vi "Write cmd queue ref.vi"(8 "error in (no error)":errorcluster, 10 "cmd queue":refnum<queue>, 11 "Plots in":refnum<class "Plots.lvclass">) -> (0 "error out":errorcluster, 3 "Plots out":refnum<class "Plots.lvclass">)   [LabVIEW 2017, in "Plots.lvclass"]
doc: "writes the reference of the commands queue to the private property. the queue is used to share data between scripts and plots."
uses:
  Plots.lvclass
  Plots.lvclass/Plots.ctl
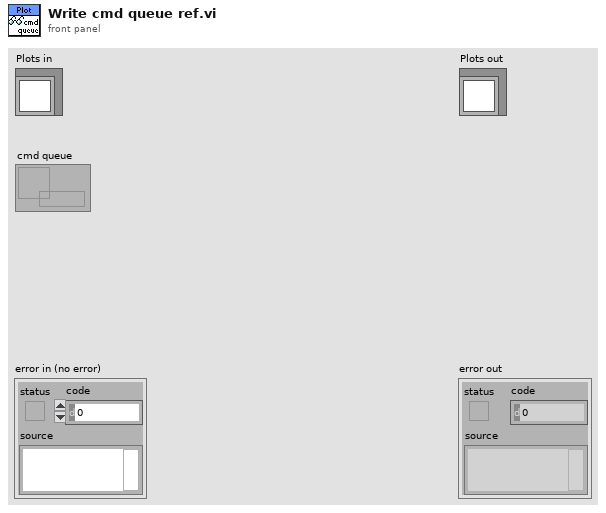
[diagram p1: front panel]
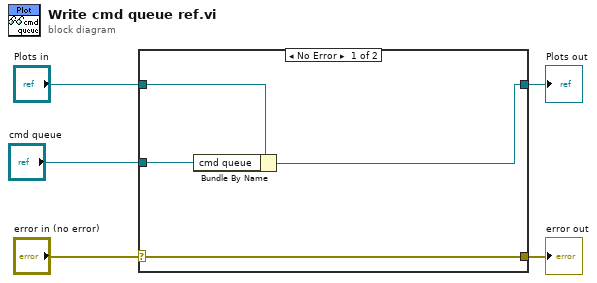
[diagram p0: block diagram]
diagram:
  n1 = case shown="No Error" "error in (no error)" {
    selector: "error in (no error)" -> [w9 w10]
    tunnel: [w9 w10] -> w4
    tunnel: [w6 w11] -> w2
    tunnel: "Plots in" -> [w7 w11]
    tunnel: "cmd queue" -> [w8 _]
    frame No Error {
      n2 = Bundle By Name(cluster=w7, "cmd queue"=w8) -> (w6:refnum<class "Plots.lvclass">)
    }
    frame Error {
    }
  }
  "error out" <- w4
  "Plots out" <- w2
